vi "Ref AVI Video Save.vi"(5 "Frame Size":u32, 6 "Channel":T1, 7 "AVI mode":T6, 8 "error in (no error)":errorcluster, 9 "AVI cluster":T2, 10 "PMT is ON?":bool, 11 "Image Pixels":i16[][](array[numeric])) -> (0 "error out":errorcluster, 2 "New split file has just been initialised":bool)   [LabVIEW 2017]
uses:
  Typedefs/AVI implementation enum.ctl
  Typedefs/AVI Refs cluster.ctl
  <vilib>/vision/Avi.llb/IMAQ AVI2 Refnum.ctl
  <vilib>/vision/Image Controls.llb/IMAQ Image.ctl
  <vilib>/vision/Avi1.llb/AviRefnum.ctl
  Typedefs/Channel Selector.ctl
panel:
  out "Number of Frames":u32
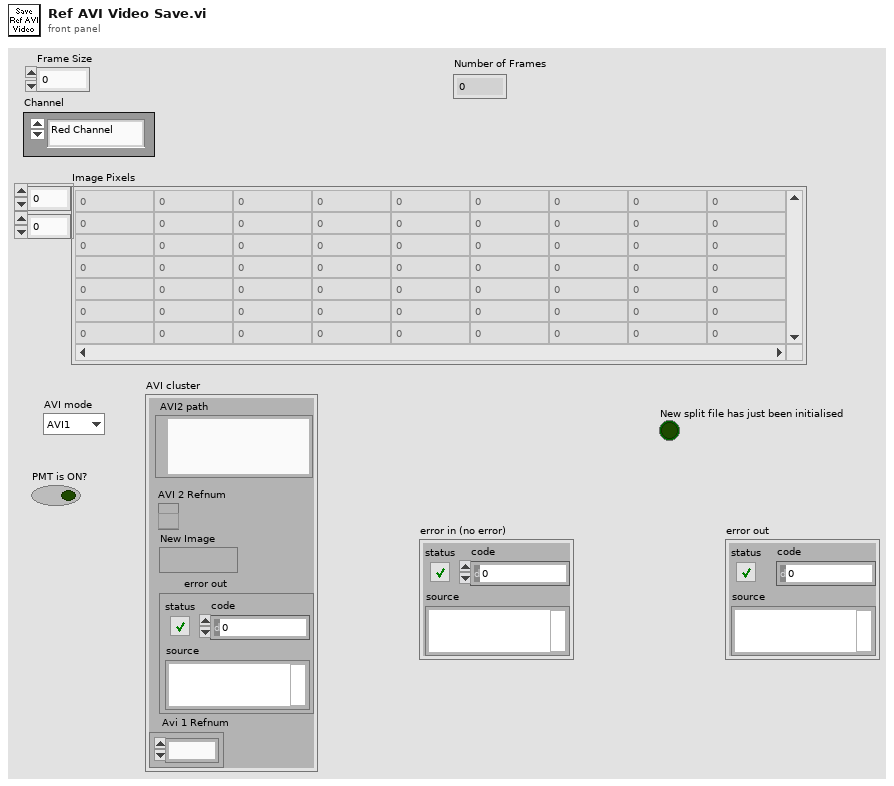
[diagram p1: front panel]
types:
  T1 = typedef "Channel Selector.ctl" = enum16{"Red Channel", "Green Channel", "Blended"}
  T2 = typedef "AVI Refs cluster.ctl" = cluster{"AVI2 path":path, "AVI 2 Refnum":T3, "New Image":T4, "error out":errorcluster, "Avi 1 Refnum":T5}
  T3 = typedef "IMAQ AVI2 Refnum.ctl" = refnum<k20>
  T4 = typedef "IMAQ Image.ctl" = refnum<image>
  T5 = typedef "AviRefnum.ctl" = refnum<k1>
  T6 = typedef "AVI implementation enum.ctl" = enum16{"AVI1", "AVI2"}
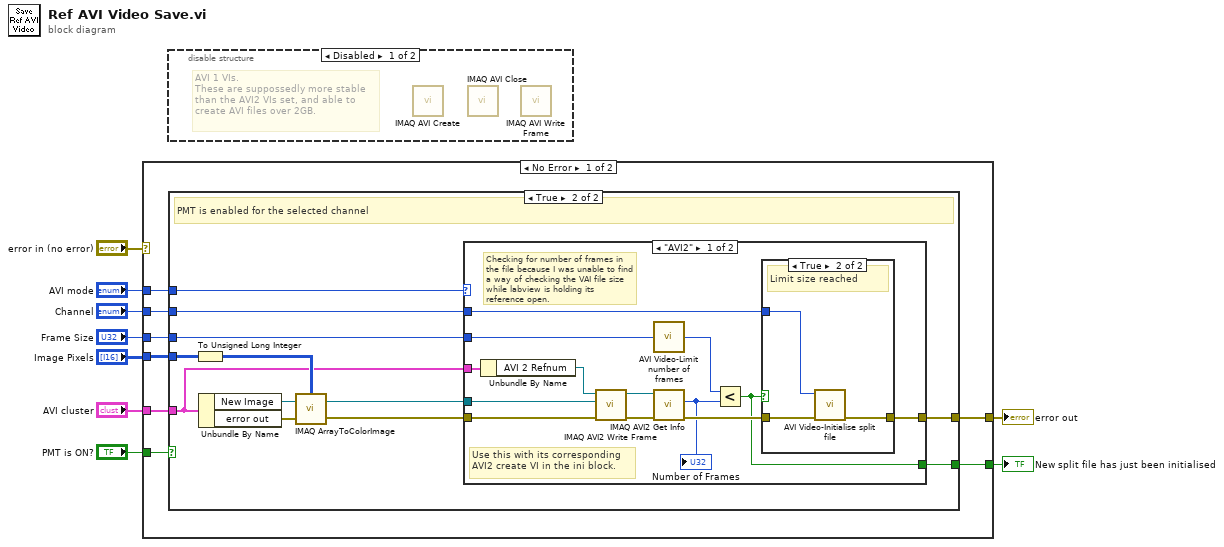
[diagram p0: block diagram]
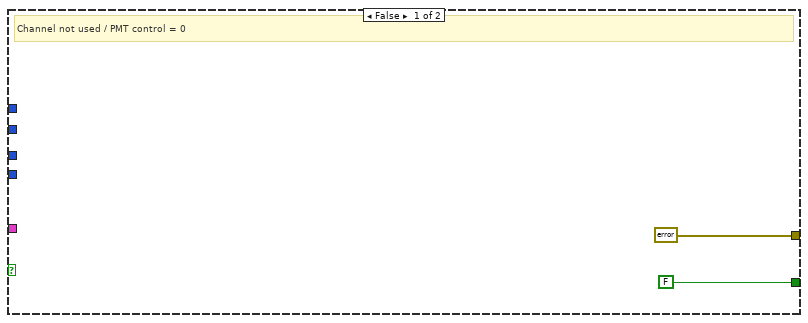
[diagram p3: hidden frame]
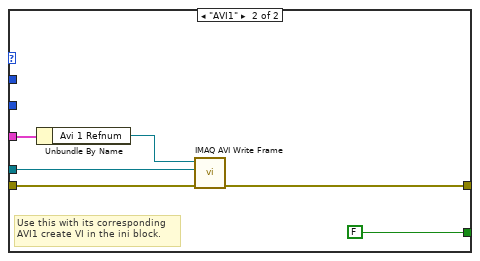
[diagram p5: hidden frame]
diagram:
  n1 = case shown="No Error" "error in (no error)" {
    tunnel: [w16 _] -> w7
    tunnel: "Image Pixels" -> [w17 _]
    tunnel: "AVI mode" -> [w15 _]
    tunnel: "AVI cluster" -> [w14 _]
    tunnel: "PMT is ON?" -> [w13 _]
    tunnel: "Channel" -> [w12 _]
    tunnel: [w11 _] -> w2
    tunnel: "Frame Size" -> [w10 _]
    frame No Error {
      n2 = case shown="True" w13 {
        tunnel: w17 -> [_ w30]
        tunnel: w14 -> [_ w23]
        tunnel: [errorcluster {"status"=FALSE, "code"=0, "source"=""} ("error out") w25] -> w16
        tunnel: w15 -> [_ w24]
        tunnel: w12 -> [_ w22]
        tunnel: [FALSE w21] -> w11
        tunnel: w10 -> [_ w20]
        frame False {
          # "Channel not used / PMT control = 0"
        }
        frame True {
          # "PMT is enabled for the selected channel"
          n3 = To Unsigned Long Integer(number=w30) -> (unsigned 32bit integer=w31:u32[][])
          n4 = Unbundle By Name(w23) -> ("New Image"=w27:T4, "error out"=w26:errorcluster)
          n5 = call "IMAQ ArrayToColorImage"("Image Pixels (U32)"=w31, "Image"=w27, "error in (no error)"=w26) -> ("Image Out"=w28:T4, "error out"=w29:errorcluster)  [unwired: 1 in, 1 out]
          n6 = case shown="\"AVI2\"" w24 {
            tunnel: w29 -> [w44 w54]
            tunnel: w28 -> [w43 w53]
            tunnel: [w40 w52] -> w25
            tunnel: w23 -> [w42 w50]
            tunnel: w22 -> [w39 _]
            tunnel: [w35 FALSE] -> w21
            tunnel: w20 -> [w32 _]
            frame "AVI2" {
              # "Checking for number of frames in the file because I was unable to find a way of checking the VAI file size while labview is holding its reference open."
              # "Use this with its corresponding\nAVI2 create VI in the ini block."
              n7 = Unbundle By Name(w42) -> ("AVI 2 Refnum"=w41:T3)
              n8 = call "IMAQ AVI2 Write Frame"("error in (no error)"=w44, "Image"=w43, "AVI Refnum"=w41) -> ("error out"=w38:errorcluster, "AVI Refnum (duplicate)"=w36:T3)  [unwired: 6 in, 1 out]
              n9 = call "AVI Video-Limit number of frames.vi"("Frame Size"=w32) -> ("Limit number of frames"=w33:u32)
              n10 = call "IMAQ AVI2 Get Info"("error in (no error)"=w38, "AVI Refnum"=w36) -> ("error out"=w37:errorcluster, "Number of Frames"=w34:u32)  [unwired: 5 in, 3 out]
              "Number of Frames" <- w34
              n11 = Less?(x=w33, y=w34) -> (x < y?=w35:bool)
              n12 = case shown="True" w35 {
                tunnel: w37 -> [w45 w48]
                tunnel: [w45 w47] -> w40
                tunnel: w39 -> [_ w46]
                frame False {
                }
                frame True {
                  # "Limit size reached"
                  n13 = call "AVI Video-Initialise split file.vi"("error in"=w48, "Channel"=w46) -> ("error out"=w47:errorcluster)  [unwired: 9 in]
                }
              }
            }
            frame "AVI1" {
              # "Use this with its corresponding\nAVI1 create VI in the ini block."
              n14 = Unbundle By Name(w50) -> ("Avi 1 Refnum"=w51:T5)
              n15 = call "IMAQ AVI Write Frame"("error in (no error)"=w54, "Image"=w53, "Avi Refnum"=w51) -> ("error out"=w52:errorcluster)  [unwired: 7 in, 1 out]
            }
          }
        }
      }
    }
    frame Error {
    }
  }
  "error out" <- w7
  "New split file has just been initialised" <- w2
  n16 = disable-structure shown="Disabled" {
    frame Disabled {
      # "AVI 1 VIs.\nThese are suppossedly more stable\nthan the AVI2 VIs set, and able to\ncreate AVI files over 2GB."
      n17 = call "IMAQ AVI Create"() -> ()  [unwired: 10 in, 2 out]
      n18 = call "IMAQ AVI Close"() -> ()  [unwired: 11 in, 1 out]
      n19 = call "IMAQ AVI Write Frame"() -> ()  [unwired: 10 in, 2 out]
    }
    frame Enabled {
    }
  }
